vi "DQMH Tester Prepare hse-appl.vi"(8 "error in":errorcluster, 11 "Real-Time App Name":string) -> (0 "error out":errorcluster, 2 "Logging Event":refnum<user-event>, 3 "Started?":bool)   [LabVIEW 2014, in "hse-dqmh.lvlib"]
doc: "If the hse-application class is not running, queries the user for the path of the containing application and instantiates the hse-appl class. Returns if it did load the class.\n\nHSE projects follow this folder structure:\n /APP-NAME_Config .......... Configuration Files\n /APP-NAME_Data .............. Measured and Other Data\n /APP-NAME_Source .......... LabVIEW Sources\n /APP-NAME ........................ Compiled Application\n\nThe hse-application:ApplicationInit.VI expects the \"APP-NAME_Source\" folder and the \"application name\", and processes these to automatically find the \"_Config\" and \"_Data\" directories.\n\nREAL-TIME: As the configuration directory on real-time systems always needs to reside at \"C:\\<Project Name>_Config\\\", and as it tedious (embedded UI) or impossible (no embedded UI) to enter the path, it can be supplied via the optional Real-Time App Name string input.\n\n\n____\nHAMPEL SOFTWARE ENGINEERING v0.7.0 (2018-07-16 18:12)"
uses:
  hse-dqmh.lvlib
  <vilib>/Hampel Software Engineering/HSE Logger/LogRecord/LogRecord.lvclass
  <vilib>/Hampel Software Engineering/HSE Logger/LogLevel.ctl
  hse-application/hse-application__GetSingleton.vi
  <vilib>/Hampel Software Engineering/HSE Logger/Handler/UserEventHandler/UserEventHandler.lvclass
  hse-application/hse-application.lvclass
  <vilib>/Hampel Software Engineering/HSE Logger/hse-logger.lvlib
panel:
  # "If the hse-application class is not running, queries the user for the path of the containing application and instantiates the hse-appl class. Returns if it did load the class.\n\nHSE projects follow this folder structure:\n    /APP-NAME_Config .......... Configuration Files\n    /APP-NAME_Data .............. Measured and Other Data\n    /APP-NAME_Source .......... LabVIEW Sources\n    /APP-NAME ........................ Compiled Application\n\nThe hse-application:ApplicationInit.VI expects the \"APP-NAME_Source\" folder and the \"application name\", and processes these to automatically find the \"_Config\" and \"_Data\" directories.\n\nREAL-TIME: As the configuration directory on real-time systems always needs to reside at \"C:\\<Project Name>_Config\\\", and as it tedious (embedded UI) or impossible (no embedded UI) to enter the path, it can be supplied via the optional Real-Time App Name string input."
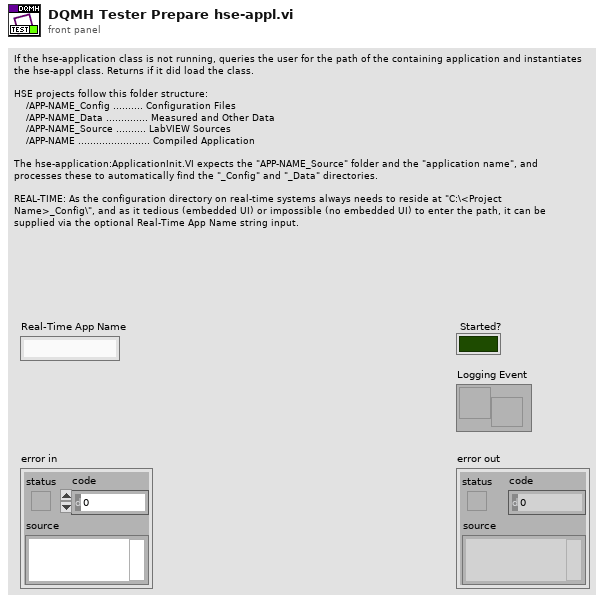
[diagram p1: front panel]
types:
  T1 = typedef "hse-logger.lvlib/LogLevel.ctl" = enum16{"DEBUG", "INFO", "WARNING", "ERROR", "CRITICAL"}
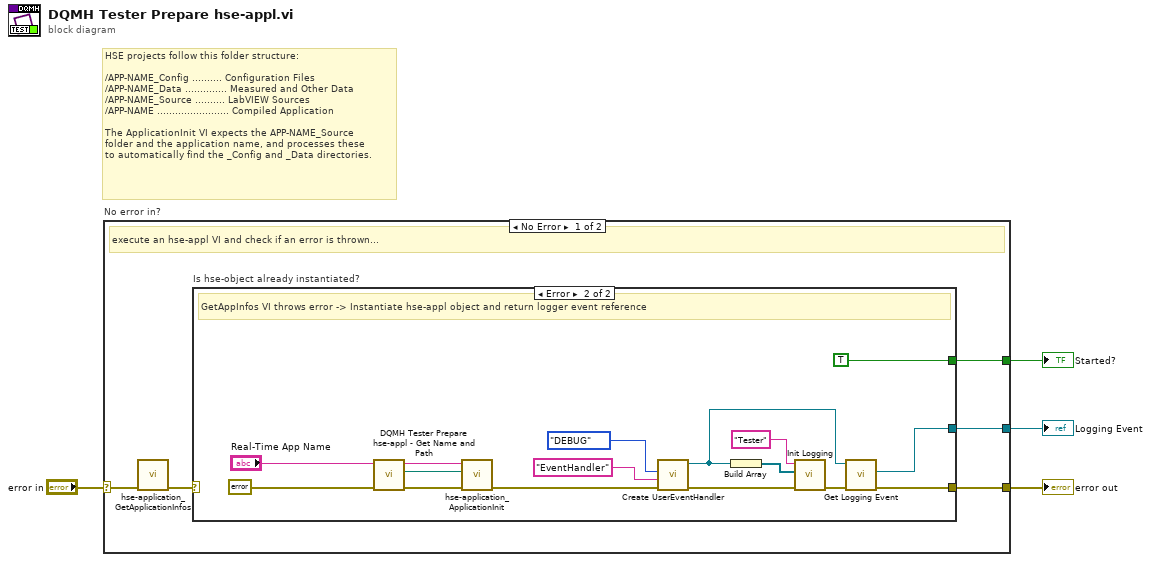
[diagram p0: block diagram]
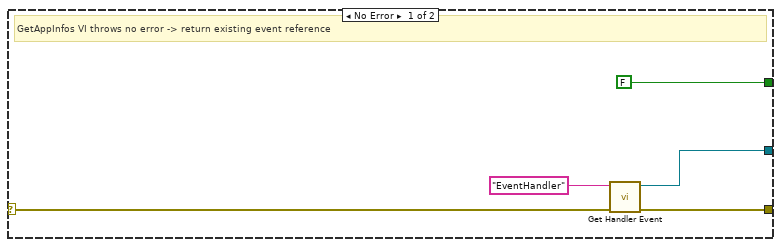
[diagram p2: hidden frame]
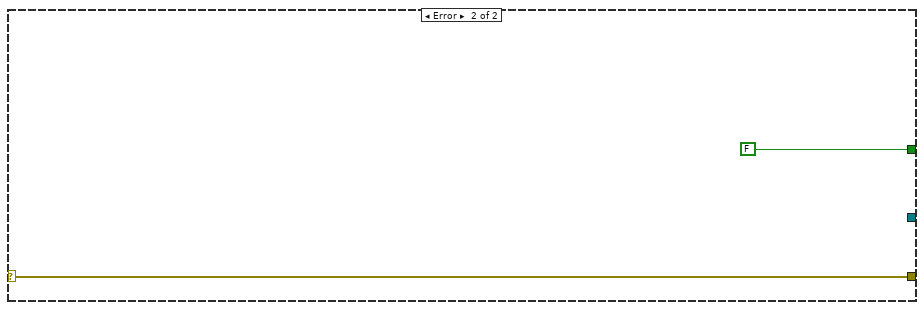
[diagram p3: hidden frame]
diagram:
  # "HSE projects follow this folder structure:\n\n/APP-NAME_Config .......... Configuration Files\n/APP-NAME_Data .............. Measured and Other Data\n/APP-NAME_Source .......... LabVIEW Sources\n/APP-NAME ........................ Compiled Application\n\nThe ApplicationInit VI expects the APP-NAME_Source\nfolder and the application name, and processes these\nto automatically find the _Config and _Data directories."
  n1 = case "No error in?" shown="No Error" "error in" {
    selector: "error in" -> [w9 w32]
    tunnel: [w6 w32] -> w4
    tunnel: [w7 FALSE] -> w2
    tunnel: [w5 _] -> w1
    frame No Error {
      # "execute an hse-appl VI and check if an error is thrown..."
      n2 = call "hse-application_GetApplicationInfos.vi"("error in"=w9) -> ("error out"=w8:errorcluster)  [unwired: 7 in, 3 out]
      n3 = case "Is hse-object already instantiated?" shown="Error" w8 {
        selector: w8 -> [w12 _]
        tunnel: [w11 w25] -> w6
        tunnel: [FALSE TRUE] -> w7
        tunnel: [w10 w24] -> w5
        frame No Error {
          # "GetAppInfos VI throws no error -> return existing event reference"
          n4 = call <vilib>:"Get Handler Event.vi"("error in"=w12, "Name"="EventHandler") -> ("error out"=w11:errorcluster, "Logging Event"=w10:refnum<user-event>)  [unwired: 8 in]
        }
        frame Error {
          # "GetAppInfos VI throws error -> Instantiate hse-appl object and return logger event reference"
          n5 = call "DQMH Tester Prepare hse-appl - Get Name and Path.vi"("error in"=errorcluster {"status"=FALSE, "code"=0, "source"=""} ("error constant"), "Real-Time App Name"="Real-Time App Name") -> ("error out"=w30:errorcluster, "Project Path"=w22:path, "Project Name"=w23:string)  [unwired: 7 in]
          n6 = call "hse-application_ApplicationInit.vi"("error in"=w30, "Project Folder"=w22, "Project Name"=w23) -> ("error out"=w19:errorcluster)  [unwired: 8 in]
          n7 = call <vilib>:"Create UserEventHandler.vi"("error in"=w19, "Name"="EventHandler", "Level"=LogLevel."DEBUG") -> ("error out"=w18:errorcluster, "UserEventHandler out"=w15:refnum<class "UserEventHandler.lvclass">)  [unwired: 7 in]
          n8 = Build Array(w15) -> (w29:refnum<class "UserEventHandler.lvclass">[])
          n9 = call <vilib>:"Init Logging.vi"("error in"=w18, "Handlers"=w29, "Name"="Tester") -> ("error out"=w26:errorcluster)  [unwired: 8 in]
          n10 = call-dynamic "Get Logging Event.vi"("error in"=w26, "UserEventHandler in"=w15) -> ("error out"=w25:errorcluster, "Logging Event"=w24:refnum<user-event>)  [unwired: 7 in, 1 out]
        }
      }
    }
    frame Error {
    }
  }
  "error out" <- w4
  "Started?" <- w2
  "Logging Event" <- w1
